vi "jMsg_TCPConnection_Update (create).vi"(8 "error in (no error)":errorcluster, 11 "Connection":T1) -> (0 "error out":errorcluster, 3 "jMsg_TCPConnection_Update":refnum<class "jMsg_TCPConnection_Update.lvclass">)   [LabVIEW 2019, in "jMsg_TCPConnection_Update.lvclass"]
doc: "This VI is used to create the jMsg\n\n\nJSMA Message Wizard 0.2.0.5\nRob Humfeld - Jet Engineering\nCopyright (c) 2020, Jet Engineering"
uses:
  jMsg_TCPConnection_Update.lvclass
  C:/Program Files/National Instruments/LabVIEW 2019/user.lib/Jet Engineering/JSMA/Libraries/jMsg Class/jMsg.lvclass
  TCPConnectionSettings STYP.ctl
  <userlib>/Jet Engineering/JSMA/Libraries/jMsg Class/jMsg.lvclass/jMsg.ctl
  jMsg_TCPConnection_Update.lvclass/jMsg_TCPConnection_Update.ctl
  <userlib>/Jet Engineering/JSMA/Libraries/Shared/JSMA_GetClassName.vi
  <vilib>/Utility/LVClass/Get LV Class Path.vi
  <userlib>/Jet Engineering/JSMA/Libraries/jMsg Class/jMsg.lvclass
panel:
  in  "jMsg_TCPConnection_Update":refnum<class "jMsg_TCPConnection_Update.lvclass">
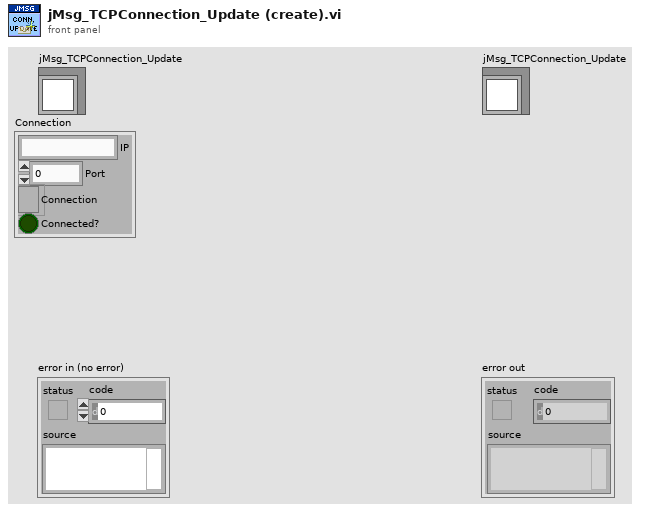
[diagram p1: front panel]
types:
  T1 = typedef "TCPConnectionSettings STYP.ctl" = cluster{"IP":string, "Port":u32, "Connection":refnum<k5>, "Connected?":bool}
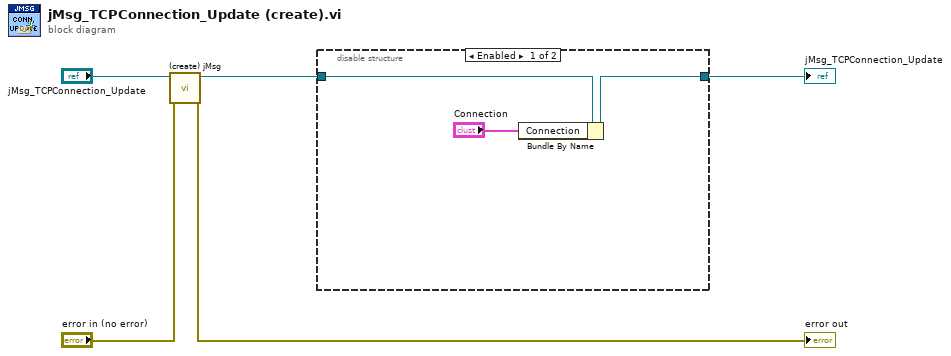
[diagram p0: block diagram]
diagram:
  n1 = call <userlib>:"(create) jMsg.vi"("error in (no error)"="error in (no error)", "jMsg in"="jMsg_TCPConnection_Update") -> ("error out"=→"error out":errorcluster, "jMsg out"=w1:refnum<class "jMsg_TCPConnection_Update.lvclass">)  [unwired: 8 in]
  n2 = disable-structure shown="Enabled" {
    disable-tunnel: w1 -> [w8 w9]
    disable-tunnel: [w7 w9] -> w5
    frame Enabled {
      n3 = Bundle By Name(cluster=w8, "Connection"="Connection") -> (w7:refnum<class "jMsg_TCPConnection_Update.lvclass">)
    }
    frame Disabled {
    }
  }
  "jMsg_TCPConnection_Update" <- w5
